vi "Get Attribute BOOL.vi"(8 "error in":errorcluster, 10 "Attribute":string, 11 "Config from XML in":refnum<class "Config from XML.lvclass">) -> (0 "error out":errorcluster, 2 "Value":bool, 3 "Config from XML out":refnum<class "Config from XML.lvclass">)   [LabVIEW 2019, in "Config from XML.lvclass"]
uses:
  Config from XML.lvclass
  Config from XML.lvclass/Config from XML.ctl
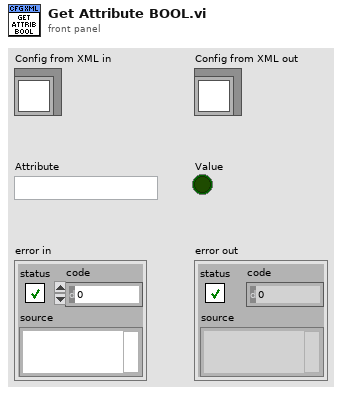
[diagram p1: front panel]
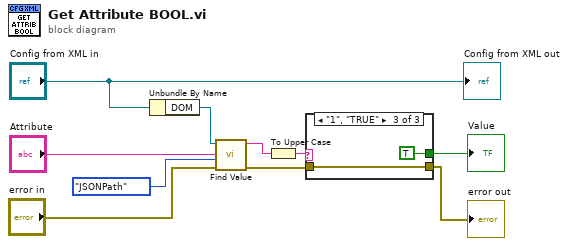
[diagram p0: block diagram]
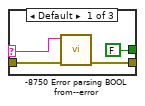
[diagram p2: hidden frame]
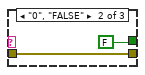
[diagram p3: hidden frame]
diagram:
  n1 = Unbundle By Name("Config from XML in") -> ("DOM"=w6:refnum<k20>)
  n2 = call "Find Value.vi"("error in"="error in", "Path Style"=enum16{"JSONPath", "XPath"}."JSONPath", "Attribute"="Attribute", "DOM"=w6) -> ("error out"=w3:errorcluster, "Value"=w2:string)  [unwired: 6 in]
  n3 = To Upper Case(1:w2) -> (0:w9:string)
  n4 = case shown="\"1\", \"TRUE\"" w9 {
    selector: w9 -> [w11 _ _]
    tunnel: [FALSE FALSE TRUE] -> w8
    tunnel: w3 -> [w14 w15 w17]
    tunnel: [w13 w15 w17] -> w7
    frame Default {
      n5 = call "-8750 Error parsing BOOL from--error.vi"("error in"=w14, "String"=w11) -> ("error out"=w13:errorcluster)  [unwired: 9 in]
    }
    frame "0", "FALSE" {
    }
    frame "1", "TRUE" {
    }
  }
  "error out" <- w7
  "Value" <- w8
  "Config from XML out" <- "Config from XML in"
